vi "AlliGator Power Law Fit from Intensity Distribution.vi"(8 "error in (no error)":errorcluster, 11 "Mouse Click Event Data":T1) -> (0 "error out":errorcluster, 1 "Message":string)   [LabVIEW 2021, in "AlliGator Lifetime & Other Parameters.lvlib"]
uses:
  AlliGator Lifetime & Other Parameters.lvlib
  Graphs/XY Graph/XY Graph Mouse Click Event Data.ctl
  Graphs/XY Graph/XY Graph Refnum.ctl
  <vilib>/Utility/miscctls.llb/LVPoint32TypeDef.ctl
  Lifetime & Other Parameters Graph Metadata.ctl
  Fits/Fit Plot Request Information.ctl
  <vilib>/Utility/miscctls.llb/LVPointDoubleTypeDef.ctl
  Fits/Fit Models.ctl
  Fits/Fit Settings.ctl
  Fits/Nonlinear Fit Method.ctl
  Fits/Ramp Type.ctl
  Fits/Residual Type.ctl
  Fits/Non-linear Fitting Algorithm.ctl
  Fits/My Fit Stopping Criteria.ctl
  Graphs/Get Plot at Mouse Click (XY Graph)/Get Plot at Mouse Click [AAC].vi
  Graphs/Graphs.lvlib
  Graphs/XY Graph/XY Graph Add-Ons.lvlib
  Fits/Fits.lvlib
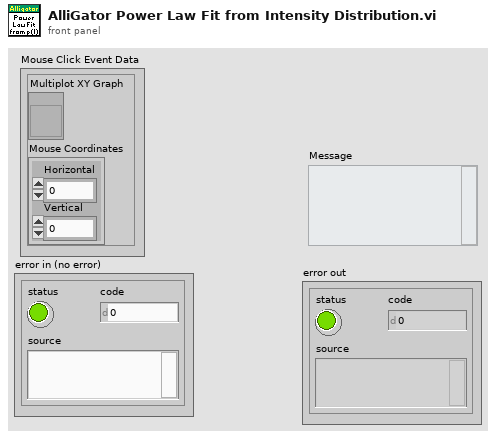
[diagram p1: front panel]
types:
  T1 = typedef "XY Graph Add-Ons.lvlib/XY Graph Mouse Click Event Data.ctl" = cluster{"Multiplot XY Graph":T2, "Mouse Coordinates":T3}
  T2 = typedef "XY Graph Add-Ons.lvlib/XY Graph Refnum.ctl" = refnum<vi>
  T3 = typedef "LVPoint32TypeDef.ctl" = cluster{"Horizontal":i32, "Vertical":i32}
  T4 = typedef "Fits.lvlib/My Fit Stopping Criteria.ctl" = cluster{"Max Iterations":i32, "Max Function Calls":i32, "Max Time":dbl[unit], "Function Tolerance":dbl, "Parameter Tolerance":dbl, "Gradient Tolerance":dbl, "Min Lambda":dbl, "Max Lambda":dbl, "Initial Tick Count":u32}
  T5 = typedef "Fits.lvlib/Fit Settings.ctl" = cluster{"Use Original Plot # Points":bool, "# Fit Plot Points":u32, "Fitting Method":T6, "Weighted Fit":bool, "Show All Fit Components":bool, "Axis Type":T7, "Show Fit Residuals":bool, "Residual Type":T8, "Fitting Algorithm":T9}
  T6 = typedef "Fits.lvlib/Nonlinear Fit Method.ctl" = enum16{"Least Square", "Least Absolute Residual", "Bisquare", "MLE"}
  T7 = typedef "Fits.lvlib/Ramp Type.ctl" = u16
  T8 = typedef "Fits.lvlib/Residual Type.ctl" = enum16{"Standard", "Normalized", "Reduced"}
  T9 = typedef "Fits.lvlib/Non-linear Fitting Algorithm.ctl" = enum16{"Levenberg-Marquardt", "Trust-Region Dogleg"}
  T10 = typedef "Fits.lvlib/Fit Models.ctl" = enum16{"Select a Fit Model...", "           Single Peak", "Gaussian", "Asymmetric Gaussian", "Lorentzian", "Asymmetric Lorentzian", "Gaussian/Lorentzian", "Lorentzian/Gaussian", "           Double Peak", "Two Gaussians", "Two Asymmetric Gaussians", "Two H-Connected Gaussians", "Two T-Connected Gaussians", "Two H-Connected Asymmetric Gaussians", "Two T-Connected Asymmetric Gaussians", "           Triple Peak", "Three Gaussians", "Three Asymmetric Gaussians", "              Decays", "1-Exponential", "IRF*PSED", "2-Exponentials", "            Power Law", "Power Law", "Power Law with Offset", "Power Law from Intensity Distribution", "               ACF", "2D Gaussian ACF", "2D Gaussian + Blinking ACF", "2D Gaussian + Flow ACF", "3D Gaussian ACF", "3D Gaussian + Blinking ACF", "             Multiplot", "2D Gaussian ACF & 2D Gaussian + Flow ACF"}
  T11 = typedef "Fits.lvlib/Fit Plot Request Information.ctl" = cluster{"XY Graph Ref":refnum<vi>, "Mouse Coordinates":T12, "Fit Model":T10, "Plot Index":i32}
  T12 = typedef "LVPointDoubleTypeDef.ctl" = cluster{"X":dbl, "Y":dbl}
  T13 = typedef "AlliGator Lifetime & Other Parameters.lvlib/Lifetime & Other Parameters Graph Metadata.ctl" = cluster{"Intensity Array":sgl[]}[]
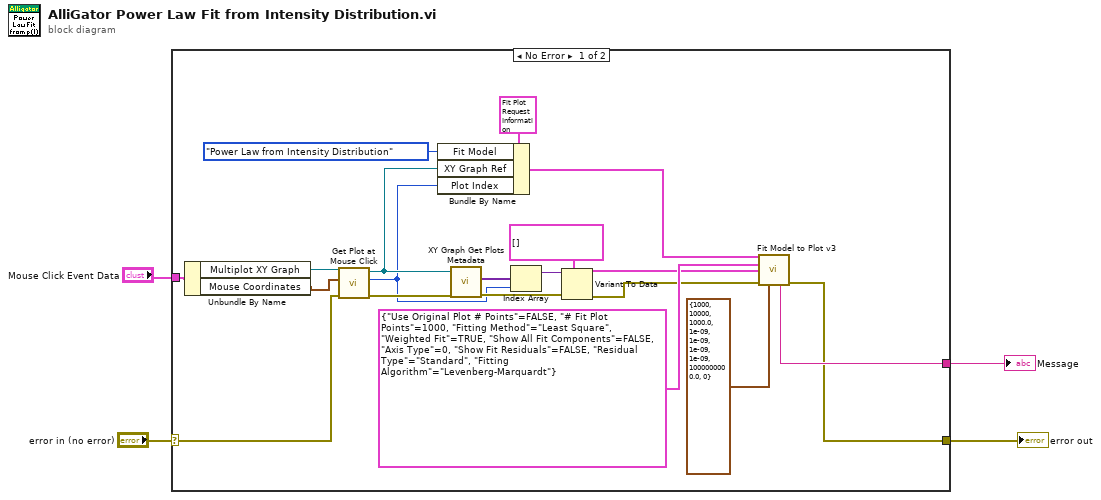
[diagram p0: block diagram]
diagram:
  n1 = case shown="No Error" "error in (no error)" {
    selector: "error in (no error)" -> [w21 w25]
    tunnel: [w5 w25] -> w4
    tunnel: "Mouse Click Event Data" -> [w24 _]
    tunnel: [w6 _] -> w1
    frame No Error {
      n2 = Unbundle By Name(w24) -> ("Multiplot XY Graph"=w23:T2, "Mouse Coordinates"=w22:T3)
      n3 = call-poly "Get Plot at Mouse Click.vi"("error in (no error)"=w21, "Mouse Click Coordinates"=w22, "XYGraph Ref"=w23) -> ("error out"=w19:errorcluster, "Plot at Coordinates"=w13:i32, "XYGraph Ref"=w14:T2)  [unwired: 2 in, 4 out]
      n4 = Bundle By Name(cluster=T11 {"XY Graph Ref"=refnum, "Mouse Coordinates"={"X"=0.0, "Y"=0.0}, "Fit Model"=enum."Power Law from Intensity Distribution", "Plot Index"=-1}, "Fit Model"=Fit_Models."Power Law from Intensity Distribution", "XY Graph Ref"=w14, "Plot Index"=w13) -> (w11:T11)
      n5 = call "XY Graph Get Plots Metadata.vi"("Error In"=w19, "XYGraph Ref"=w14) -> ("Error Out"=w18:errorcluster, "Plots Metadata"=w20:variant[])  [unwired: 6 in, 2 out]
      n6 = Index Array(array=w20, index=w13) -> (element=w17:variant)
      n7 = Variant To Data(error in=w18, type=T13 [] ("Lifetime & Other Parameters Graph Metadata"), Variant=w17) -> (data=w9:T13, error out=w8:errorcluster)
      n8 = call "Fit Model to Plot v3.vi"("Fit Plot Information"=w11, "Fit Settings"=T5 {"Use Original Plot # Points"=FALSE, "# Fit Plot Points"=1000, "Fitting Method"=enum."Least Square", "Weighted Fit"=TRUE, "Show All Fit Components"=FALSE, "Axis Type"=0, "Show Fit Residuals"=FALSE, "Residual Type"=enum."Standard", "Fitting Algorithm"=enum."Levenberg-Marquardt"}, "Additional Parameters (in)"=w9, "error in (no error)"=w8, "Termination Criteria"=T4 {"Max Iterations"=1000, "Max Function Calls"=10000, "Max Time"=1000.0, "Function Tolerance"=1e-09, "Parameter Tolerance"=1e-09, "Gradient Tolerance"=1e-09, "Min Lambda"=1e-09, "Max Lambda"=1000000000.0, "Initial Tick Count"=0}) -> ("Fit Result String"=w6:string, "error out"=w5:errorcluster)  [unwired: 2 in, 7 out]
    }
    frame Error {
    }
  }
  "error out" <- w4
  "Message" <- w1
